vi "Methods to Method Info.vi"(10 "Class":string, 11 "Methods from Node":T2(array[cluster])) -> (2 "Methods for Tree":T1(array[cluster]), 3 "Methods[]":T3(array[cluster]))   [LabVIEW 2023] (continued)
"Class Name (localized)"="VI"}, "Method Info"={"Unique ID string"="42a", "Data name"="Transaction.Fail", "Short name (localized)"="Transaction.Fail", "Long name (localized)"="Transaction:Fail"}, "Method Flags"={"IsDeprecated"=FALSE, "IsPrivate"=FALSE, "IsScripting"=TRUE, "IsNotInRun-Time"=TRUE}, "Divider"=FALSE}, {"Class Info"={"Unique ID string"="2", "Parent ID string"="", "Class Name (unlocalized)"="VI", "Class Name (localized)"="VI"}, "Method Info"={"Unique ID string"="42b", "Data name"="VI Strings.Export Private", "Short name (localized)"="VI Strings.Export Private", "Long name (localized)"="VI Strings:Export Private"}, "Method Flags"={"IsDeprecated"=FALSE, "IsPrivate"=TRUE, "IsScripting"=FALSE, "IsNotInRun-Time"=TRUE}, "Divider"=FALSE}, {"Class Info"={"Unique ID string"="2", "Parent ID string"="", "Class Name (unlocalized)"="VI", "Class Name (localized)"="VI"}, "Method Info"={"Unique ID string"="42c", "Data name"="BD.Get Image Scaled", "Short name (localized)"="BD.Get Image Scaled", "Long name (localized)"="Block Diagram:Get Image Scaled"}, "Method Flags"={"IsDeprecated"=FALSE, "IsPrivate"=FALSE, "IsScripting"=FALSE, "IsNotInRun-Time"=TRUE}, "Divider"=FALSE}, {"Class Info"={"Unique ID string"="2", "Parent ID string"="", "Class Name (unlocalized)"="VI", "Class Name (localized)"="VI"}, "Method Info"={"Unique ID string"="42d", "Data name"="Get Conpane Image", "Short name (localized)"="Get Conpane Image", "Long name (localized)"="Get Conpane Image"}, "Method Flags"={"IsDeprecated"=FALSE, "IsPrivate"=FALSE, "IsScripting"=TRUE, "IsNotInRun-Time"=FALSE}, "Divider"=FALSE}, {"Class Info"={"Unique ID string"="2", "Parent ID string"="", "Class Name (unlocalized)"="VI", "Class Name (localized)"="VI"}, "Method Info"={"Unique ID string"="42e", "Data name"="RP.Lock Control", "Short name (localized)"="RP.Lock Control", "Long name (localized)"="Remote Panel:Lock Control"}, "Method Flags"={"IsDeprecated"=FALSE, "IsPrivate"=FALSE, "IsScripting"=FALSE, "IsNotInRun-Time"=FALSE}, "Divider"=FALSE}, {"Class Info"={"Unique ID string"="2", "Parent ID string"="", "Class Name (unlocalized)"="VI", "Class Name (localized)"="VI"}, "Method Info"={"Unique ID string"="42f", "Data name"="RP.Unlock Control", "Short name (localized)"="RP.Unlock Control", "Long name (localized)"="Remote Panel:Unlock Control"}, "Method Flags"={"IsDeprecated"=FALSE, "IsPrivate"=FALSE, "IsScripting"=FALSE, "IsNotInRun-Time"=FALSE}, "Divider"=FALSE}, {"Class Info"={"Unique ID string"="2", "Parent ID string"="", "Class Name (unlocalized)"="VI", "Class Name (localized)"="VI"}, "Method Info"={"Unique ID string"="430", "Data name"="RP.Client Connections", "Short name (localized)"="RP.Client Connections", "Long name (localized)"="Remote Panel:Client Connections"}, "Method Flags"={"IsDeprecated"=FALSE, "IsPrivate"=FALSE, "IsScripting"=FALSE, "IsNotInRun-Time"=FALSE}, "Divider"=FALSE}, {"Class Info"={"Unique ID string"="2", "Parent ID string"="", "Class Name (unlocalized)"="VI", "Class Name (localized)"="VI"}, "Method Info"={"Unique ID string"="431", "Data name"="RP.Close Connection To Client", "Short name (localized)"="RP.Close Connection To Client", "Long name (localized)"="Remote Panel:Close Connection To Client"}, "Method Flags"={"IsDeprecated"=FALSE, "IsPrivate"=FALSE, "IsScripting"=FALSE, "IsNotInRun-Time"=FALSE}, "Divider"=FALSE}, {"Class Info"={"Unique ID string"="2", "Parent ID string"="", "Class Name (unlocalized)"="VI", "Class Name (localized)"="VI"}, "Method Info"={"Unique ID string"="432", "Data name"="User Edits.Allow", "Short name (localized)"="User Edits.Allow", "Long name (localized)"="User Edits:Allow"}, "Method Flags"={"IsDeprecated"=FALSE, "IsPrivate"=TRUE, "IsScripting"=FALSE, "IsNotInRun-Time"=FALSE}, "Divider"=FALSE}, {"Class Info"={"Unique ID string"="2", "Parent ID string"="", "Class Name (unlocalized)"="VI", "Class Name (localized)"="VI"}, "Method Info"={"Unique ID string"="433", "Data name"="User Edits.Block", "Short name (localized)"="User Edits.Block", "Long name (localized)"="User Edits:Block"}, "Method Flags"={"IsDeprecated"=FALSE, "IsPrivate"=TRUE, "IsScripting"=FALSE, "IsNotInRun-Time"=FALSE}, "Divider"=FALSE}, {"Class Info"={"Unique ID string"="2", "Parent ID string"="", "Class Name (unlocalized)"="VI", "Class Name (localized)"="VI"}, "Method Info"={"Unique ID string"="434", "Data name"="FP.Set Close If Lonely", "Short name (localized)"="FP.Set Close If Lonely", "Long name (localized)"="Front Panel:Set Close If Lonely"}, "Method Flags"={"IsDeprecated"=FALSE, "IsPrivate"=TRUE, "IsScripting"=TRUE, "IsNotInRun-Time"=FALSE}, "Divider"=FALSE}, {"Class Info"={"Unique ID string"="2", "Parent ID string"="", "Class Name (unlocalized)"="VI", "Class Name (localized)"="VI"}, "Method Info"={"Unique ID string"="435", "Data name"="VI Hier.Get User GUID", "Short name (localized)"="VI Hier.Get User GUID", "Long name (localized)"="VI Hierarchy:Get User GUID"}, "Method Flags"={"IsDeprecated"=FALSE, "IsPrivate"=TRUE, "IsScripting"=FALSE, "IsNotInRun-Time"=FALSE}, "Divider"=FALSE}, {"Class Info"={"Unique ID string"="2", "Parent ID string"="", "Class Name (unlocalized)"="VI", "Class Name (localized)"="VI"}, "Method Info"={"Unique ID string"="437", "Data name"="Cause Type Propagation", "Short name (localized)"="Cause Type Propagation", "Long name (localized)"="Cause Type Propagation"}, "Method Flags"={"IsDeprecated"=FALSE, "IsPrivate"=TRUE, "IsScripting"=TRUE, "IsNotInRun-Time"=FALSE}, "Divider"=FALSE}, {"Class Info"={"Unique ID string"="2", "Parent ID string"="", "Class Name (unlocalized)"="VI", "Class Name (localized)"="VI"}, "Method Info"={"Unique ID string"="438", "Data name"="FP.Open", "Short name (localized)"="FP.Open", "Long name (localized)"="Front Panel:Open"}, "Method Flags"={"IsDeprecated"=FALSE, "IsPrivate"=FALSE, "IsScripting"=FALSE, "IsNotInRun-Time"=FALSE}, "Divider"=FALSE}, {"Class Info"={"Unique ID string"="2", "Parent ID string"="", "Class Name (unlocalized)"="VI", "Class Name (localized)"="VI"}, "Method Info"={"Unique ID string"="439", "Data name"="BD.Set Mod", "Short name (localized)"="BD.Set Mod", "Long name (localized)"="Block Diagram:Set Mod"}, "Method Flags"={"IsDeprecated"=FALSE, "IsPrivate"=TRUE, "IsScripting"=FALSE, "IsNotInRun-Time"=TRUE}, "Divider"=FALSE}, {"Class Info"={"Unique ID string"="2", "Parent ID string"="", "Class Name (unlocalized)"="VI", "Class Name (localized)"="VI"}, "Method Info"={"Unique ID string"="43a", "Data name"="FP.Set Mod", "Short name (localized)"="FP.Set Mod", "Long name (localized)"="Front Panel:Set Mod"}, "Method Flags"={"IsDeprecated"=FALSE, "IsPrivate"=TRUE, "IsScripting"=FALSE, "IsNotInRun-Time"=TRUE}, "Divider"=FALSE}, {"Class Info"={"Unique ID string"="2", "Parent ID string"="", "Class Name (unlocalized)"="VI", "Class Name (localized)"="VI"}, "Method Info"={"Unique ID string"="43b", "Data name"="Adapt Nodes Private", "Short name (localized)"="Adapt Nodes Private", "Long name (localized)"="Adapt Nodes Private"}, "Method Flags"={"IsDeprecated"=FALSE, "IsPrivate"=TRUE, "IsScripting"=TRUE, "IsNotInRun-Time"=TRUE}, "Divider"=FALSE}, {"Class Info"={"Unique ID string"="2", "Parent ID string"="", "Class Name (unlocalized)"="VI", "Class Name (localized)"="VI"}, "Method Info"={"Unique ID string"="43c", "Data name"="Adapt Nodes", "Short name (localized)"="Adapt Nodes", "Long name (localized)"="Adapt Nodes"}, "Method Flags"={"IsDeprecated"=FALSE, "IsPrivate"=FALSE, "IsScripting"=TRUE, "IsNotInRun-Time"=TRUE}, "Divider"=FALSE}, {"Class Info"={"Unique ID string"="2", "Parent ID string"="", "Class Name (unlocalized)"="VI", "Class Name (localized)"="VI"}, "Method Info"={"Unique ID string"="43e", "Data name"="Synch In All Contexts", "Short name (localized)"="Synch In All Contexts", "Long name (localized)"="Synchronize In All Contexts"}, "Method Flags"={"IsDeprecated"=FALSE, "IsPrivate"=TRUE, "IsScripting"=FALSE, "IsNotInRun-Time"=FALSE}, "Divider"=FALSE}, {"Class Info"={"Unique ID string"="2", "Parent ID string"="", "Class Name (unlocalized)"="VI", "Class Name (localized)"="VI"}, "Method Info"={"Unique ID string"="43f", "Data name"="Enter Text", "Short name (localized)"="Enter Text", "Long name (localized)"="Enter Text"}, "Method Flags"={"IsDeprecated"=FALSE, "IsPrivate"=TRUE, "IsScripting"=FALSE, "IsNotInRun-Time"=FALSE}, "Divider"=FALSE}, {"Class Info"={"Unique ID string"="2", "Parent ID string"="", "Class Name (unlocalized)"="VI", "Class Name (localized)"="VI"}, "Method Info"={"Unique ID string"="440", "Data name"="Gen C Code Variant", "Short name (localized)"="Gen C Code Variant", "Long name (localized)"="Generate C Code Variant"}, "Method Flags"={"IsDeprecated"=FALSE, "IsPrivate"=TRUE, "IsScripting"=FALSE, "IsNotInRun-Time"=FALSE}, "Divider"=FALSE}, {"Class Info"={"Unique ID string"="2", "Parent ID string"="", "Class Name (unlocalized)"="VI", "Class Name (localized)"="VI"}, "Method Info"={"Unique ID string"="441", "Data name"="FP.Center", "Short name (localized)"="FP.Center", "Long name (localized)"="Front Panel:Center"}, "Method Flags"={"IsDeprecated"=FALSE, "IsPrivate"=FALSE, "IsScripting"=FALSE, "IsNotInRun-Time"=FALSE}, "Divider"=FALSE}, {"Class Info"={"Unique ID string"="2", "Parent ID string"="", "Class Name (unlocalized)"="VI", "Class Name (localized)"="VI"}, "Method Info"={"Unique ID string"="443", "Data name"="Create from Reference", "Short name (localized)"="Create from Reference", "Long name (localized)"="Create from Reference"}, "Method Flags"={"IsDeprecated"=FALSE, "IsPrivate"=FALSE, "IsScripting"=TRUE, "IsNotInRun-Time"=TRUE}, "Divider"=FALSE}, {"Class Info"={"Unique ID string"="2", "Parent ID string"="", "Class Name (unlocalized)"="VI", "Class Name (localized)"="VI"}, "Method Info"={"Unique ID string"="445", "Data name"="FP.Run-Time Pos.Get", "Short name (localized)"="FP.Run-Time Pos.Get", "Long name (localized)"="Front Panel:Run-Time Position:Get Position"}, "Method Flags"={"IsDeprecated"=FALSE, "IsPrivate"=FALSE, "IsScripting"=FALSE, "IsNotInRun-Time"=FALSE}, "Divider"=FALSE}, {"Class Info"={"Unique ID string"="2", "Parent ID string"="", "Class Name (unlocalized)"="VI", "Class Name (localized)"="VI"}, "Method Info"={"Unique ID string"="446", "Data name"="FP.Run-Time Pos.Unchanged", "Short name (localized)"="FP.Run-Time Pos.Unchanged", "Long name (localized)"="Front Panel:Run-Time Position:Unchanged"}, "Method Flags"={"IsDeprecated"=FALSE, "IsPrivate"=FALSE, "IsScripting"=FALSE, "IsNotInRun-Time"=FALSE}, "Divider"=FALSE}, {"Class Info"={"Unique ID string"="2", "Parent ID string"="", "Class Name (unlocalized)"="VI", "Class Name (localized)"="VI"}, "Method Info"={"Unique ID string"="447", "Data name"="FP.Run-Time Position.Centered", "Short name (localized)"="FP.Run-Time Position.Centered", "Long name (localized)"="Front Panel:Run-Time Position:Centered"}, "Method Flags"={"IsDeprecated"=FALSE, "IsPrivate"=FALSE, "IsScripting"=FALSE, "IsNotInRun-Time"=FALSE}, "Divider"=FALSE}, {"Class Info"={"Unique ID string"="2", "Parent ID string"="", "Class Name (unlocalized)"="VI", "Class Name (localized)"="VI"}, "Method Info"={"Unique ID string"="448", "Data name"="FP.Run-Time Position.Maximized", "Short name (localized)"="FP.Run-Time Position.Maximized", "Long name (localized)"="Front Panel:Run-Time Position:Maximized"}, "Method Flags"={"IsDeprecated"=FALSE, "IsPrivate"=FALSE, "IsScripting"=FALSE, "IsNotInRun-Time"=FALSE}, "Divider"=FALSE}, {"Class Info"={"Unique ID string"="2", "Parent ID string"="", "Class Name (unlocalized)"="VI", "Class Name (localized)"="VI"}, "Method Info"={"Unique ID string"="449", "Data name"="FP.Run-Time Position.Minimized", "Short name (localized)"="FP.Run-Time Position.Minimized", "Long name (localized)"="Front Panel:Run-Time Position:Minimized"}, "Method Flags"={"IsDeprecated"=FALSE, "IsPrivate"=FALSE, "IsScripting"=FALSE, "IsNotInRun-Time"=FALSE}, "Divider"=FALSE}, {"Class Info"={"Unique ID string"="2", "Parent ID string"="", "Class Name (unlocalized)"="VI", "Class Name (localized)"="VI"}, "Method Info"={"Unique ID string"="44a", "Data name"="FP.Run-Time Position.Custom", "Short name (localized)"="FP.Run-Time Position.Custom", "Long name (localized)"="Front Panel:Run-Time Position:Custom"}, "Method Flags"={"IsDeprecated"=FALSE, "IsPrivate"=FALSE, "IsScripting"=FALSE, "IsNotInRun-Time"=FALSE}, "Divider"=FALSE}, {"Class Info"={"Unique ID string"="2", "Parent ID string"="", "Class Name (unlocalized)"="VI", "Class Name (localized)"="VI"}, "Method Info"={"Unique ID string"="44b", "Data name"="DisconnectFromLibrary", "Short name (localized)"="DisconnectFromLibrary", "Long name (localized)"="Disconnect From Library"}, "Method Flags"={"IsDeprecated"=FALSE, "IsPrivate"=FALSE, "IsScripting"=FALSE, "IsNotInRun-Time"=TRUE}, "Divider"=FALSE}, {"Class Info"={"Unique ID string"="2", "Parent ID string"="", "Class Name (unlocalized)"="VI", "Class Name (localized)"="VI"}, "Method Info"={"Unique ID string"="44d", "Data name"="Replicate Conpane", "Short name (localized)"="Replicate Conpane", "Long name (localized)"="Replicate Conpane"}, "Method Flags"={"IsDeprecated"=FALSE, "IsPrivate"=FALSE, "IsScripting"=TRUE, "IsNotInRun-Time"=FALSE}, "Divider"=FALSE}, {"Class Info"={"Unique ID string"="2", "Parent ID string"="", "Class Name (unlocalized)"="VI", "Class Name (localized)"="VI"}, "Method Info"={"Unique ID string"="44e", "Data name"="AddASPending", "Short name (localized)"="AddASPending", "Long name (localized)"="Add To AutoSave Pending List"}, "Method Flags"={"IsDeprecated"=FALSE, "IsPrivate"=TRUE, "IsScripting"=FALSE, "IsNotInRun-Time"=TRUE}, "Divider"=FALSE}, {"Class Info"={"Unique ID string"="2", "Parent ID string"="", "Class Name (unlocalized)"="VI", "Class Name (localized)"="VI"}, "Method Info"={"Unique ID string"="44f", "Data name"="RemoveBreakpoints", "Short name (localized)"="RemoveBreakpoints", "Long name (localized)"="Remove Breakpoints"}, "Method Flags"={"IsDeprecated"=FALSE, "IsPrivate"=TRUE, "IsScripting"=TRUE, "IsNotInRun-Time"=FALSE}, "Divider"=FALSE}, {"Class Info"={"Unique ID string"="2", "Parent ID string"="", "Class Name (unlocalized)"="VI", "Class Name (localized)"="VI"}, "Method Info"={"Unique ID string"="451", "Data name"="Save.Instrument(NoSync)", "Short name (localized)"="Save.Instrument(NoSync)", "Long name (localized)"="Save:Instrument (No Sync)"}, "Method Flags"={"IsDeprecated"=FALSE, "IsPrivate"=TRUE, "IsScripting"=FALSE, "IsNotInRun-Time"=TRUE}, "Divider"=FALSE}, {"Class Info"={"Unique ID string"="2", "Parent ID string"="", "Class Name (unlocalized)"="VI", "Class Name (localized)"="VI"}, "Method Info"={"Unique ID string"="452", "Data name"="Get Errors", "Short name (localized)"="Get Errors", "Long name (localized)"="Get Errors"}, "Method Flags"={"IsDeprecated"=FALSE, "IsPrivate"=TRUE, "IsScripting"=TRUE, "IsNotInRun-Time"=FALSE}, "Divider"=FALSE}, {"Class Info"={"Unique ID string"="2", "Parent ID string"="", "Class Name (unlocalized)"="VI", "Class Name (localized)"="VI"}, "Method Info"={"Unique ID string"="453", "Data name"="Tag.Get Tag Names", "Short name (localized)"="Tag.Get Tag Names", "Long name (localized)"="Tag:Get Names"}, "Method Flags"={"IsDeprecated"=FALSE, "IsPrivate"=TRUE, "IsScripting"=FALSE, "IsNotInRun-Time"=FALSE}, "Divider"=FALSE}, {"Class Info"={"Unique ID string"="2", "Parent ID string"="", "Class Name (unlocalized)"="VI", "Class Name (localized)"="VI"}, "Method Info"={"Unique ID string"="454", "Data name"="GiveTemporaryUnsavedName", "Short name (localized)"="GiveTemporaryUnsavedName", "Long name (localized)"="Give Temporary Unsaved Name"}, "Method Flags"={"IsDeprecated"=FALSE, "IsPrivate"=TRUE, "IsScripting"=FALSE, "IsNotInRun-Time"=TRUE}, "Divider"=FALSE}, {"Class Info"={"Unique ID string"="2", "Parent ID string"="", "Class Name (unlocalized)"="VI", "Class Name (localized)"="VI"}, "Method Info"={"Unique ID string"="455", "Data name"="SetOnlineEdit", "Short name (localized)"="SetOnlineEdit", "Long name (localized)"="Set Online Edit"}, "Method Flags"={"IsDeprecated"=FALSE, "IsPrivate"=TRUE, "IsScripting"=FALSE, "IsNotInRun-Time"=FALSE}, "Divider"=FALSE}, {"Class Info"={"Unique ID string"="2", "Parent ID string"="", "Class Name (unlocalized)"="VI", "Class Name (localized)"="VI"}, "Method Info"={"Unique ID string"="457", "Data name"="CtlVIApplyChanges", "Short name (localized)"="CtlVIApplyChanges", "Long name (localized)"="Control VI Apply Changes"}, "Method Flags"={"IsDeprecated"=FALSE, "IsPrivate"=TRUE, "IsScripting"=FALSE, "IsNotInRun-Time"=FALSE}, "Divider"=FALSE}, {"Class Info"={"Unique ID string"="2", "Parent ID string"="", "Class Name (unlocalized)"="VI", "Class Name (localized)"="VI"}, "Method Info"={"Unique ID string"="458", "Data name"="Set Path", "Short name (localized)"="Set Path", "Long name (localized)"="Set Path"}, "Method Flags"={"IsDeprecated"=FALSE, "IsPrivate"=TRUE, "IsScripting"=FALSE, "IsNotInRun-Time"=TRUE}, "Divider"=FALSE}, {"Class Info"={"Unique ID string"="2", "Parent ID string"="", "Class Name (unlocalized)"="VI", "Class Name (localized)"="VI"}, "Method Info"={"Unique ID string"="459", "Data name"="Set Filename", "Short name (localized)"="Set Filename", "Long name (localized)"="Set Filename"}, "Method Flags"={"IsDeprecated"=FALSE, "IsPrivate"=TRUE, "IsScripting"=TRUE, "IsNotInRun-Time"=FALSE}, "Divider"=FALSE}, {"Class Info"={"Unique ID string"="2", "Parent ID string"="", "Class Name (unlocalized)"="VI", "Class Name (localized)"="VI"}, "Method Info"={"Unique ID string"="45a", "Data name"="Save.CopyAsSystem", "Short name (localized)"="Save.CopyAsSystem", "Long name (localized)"="Save:Copy As System"}, "Method Flags"={"IsDeprecated"=FALSE, "IsPrivate"=TRUE, "IsScripting"=TRUE, "IsNotInRun-Time"=FALSE}, "Divider"=FALSE}, {"Class Info"={"Unique ID string"="2", "Parent ID string"="", "Class Name (unlocalized)"="VI", "Class Name (localized)"="VI"}, "Method Info"={"Unique ID string"="45c", "Data name"="Save.Instrument and Callers Debug", "Short name (localized)"="Save.Instrument and Callers Debug", "Long name (localized)"="Save:Instrument and Callers Debug"}, "Method Flags"={"IsDeprecated"=FALSE, "IsPrivate"=TRUE, "IsScripting"=FALSE, "IsNotInRun-Time"=TRUE}, "Divider"=FALSE}, {"Class Info"={"Unique ID string"="2", "Parent ID string"="", "Class Name (unlocalized)"="VI", "Class Name (localized)"="VI"}, "Method Info"={"Unique ID string"="45d", "Data name"="InvokeBuiltinMenuItem (Not Implemented)", "Short name (localized)"="InvokeBuiltinMenuItem (Not Implemented)", "Long name (localized)"="Invoke Built in Menu Item (Not Implemented)"}, "Method Flags"={"IsDeprecated"=FALSE, "IsPrivate"=TRUE, "IsScripting"=FALSE, "IsNotInRun-Time"=FALSE}, "Divider"=FALSE}, {"Class Info"={"Unique ID string"="2", "Parent ID string"="", "Class Name (unlocalized)"="VI", "Class Name (localized)"="VI"}, "Method Info"={"Unique ID string"="45e", "Data name"="BeginScript (Not Implemented)", "Short name (localized)"="BeginScript (Not Implemented)", "Long name (localized)"="Begin Scripting (Not Implemented)"}, "Method Flags"={"IsDeprecated"=FALSE, "IsPrivate"=TRUE, "IsScripting"=TRUE, "IsNotInRun-Time"=FALSE}, "Divider"=FALSE}, {"Class Info"={"Unique ID string"="2", "Parent ID string"="", "Class Name (unlocalized)"="VI", "Class Name (localized)"="VI"}, "Method Info"={"Unique ID string"="45f", "Data name"="EndScript (Not Implemented)", "Short name (localized)"="EndScript (Not Implemented)", "Long name (localized)"="End Scripting (Not Implemented)"}, "Method Flags"={"IsDeprecated"=FALSE, "IsPrivate"=TRUE, "IsScripting"=TRUE, "IsNotInRun-Time"=FALSE}, "Divider"=FALSE}, {"Class Info"={"Unique ID string"="2", "Parent ID string"="", "Class Name (unlocalized)"="VI", "Class Name (localized)"="VI"}, "Method Info"={"Unique ID string"="460", "Data name"="MoveObjects", "Short name (localized)"="MoveObjects", "Long name (localized)"="Move Objects"}, "Method Flags"={"IsDeprecated"=FALSE, "IsPrivate"=FALSE, "IsScripting"=TRUE, "IsNotInRun-Time"=TRUE}, "Divider"=FALSE}, {"Class Info"={"Unique ID string"="2", "Parent ID string"="", "Class Name (unlocalized)"="VI", "Class Name (localized)"="VI"}, "Method Info"={"Unique ID string"="461", "Data name"="GetMenuItemState (Not Implemented)", "Short name (localized)"="GetMenuItemState (Not Implemented)", "Long name (localized)"="Get Menu Item State (Not Implemented)"}, "Method Flags"={"IsDeprecated"=FALSE, "IsPrivate"=TRUE, "IsScripting"=FALSE, "IsNotInRun-Time"=FALSE}, "Divider"=FALSE}, {"Class Info"={"Unique ID string"="2", "Parent ID string"="", "Class Name (unlocalized)"="VI", "Class Name (localized)"="VI"}, "Method Info"={"Unique ID string"="462", "Data name"="SuppressBackup (Not Implemented)", "Short name (localized)"="SuppressBackup (Not Implemented)", "Long name (localized)"="Backup:Suppress (Not Implemented)"}, "Method Flags"={"IsDeprecated"=FALSE, "IsPrivate"=TRUE, "IsScripting"=FALSE, "IsNotInRun-Time"=FALSE}, "Divider"=FALSE}, {"Class Info"={"Unique ID string"="2", "Parent ID string"="", "Class Name (unlocalized)"="VI", "Class Name (localized)"="VI"}, "Method Info"={"Unique ID string"="463", "Data name"="UnsuppressBackup (Not Implemented)", "Short name (localized)"="UnsuppressBackup (Not Implemented)", "Long name (localized)"="Backup:Unsuppress (Not Implemented)"}, "Method Flags"={"IsDeprecated"=FALSE, "IsPrivate"=TRUE, "IsScripting"=FALSE, "IsNotInRun-Time"=FALSE}, "Divider"=FALSE}, {"Class Info"={"Unique ID string"="2", "Parent ID string"="", "Class Name (unlocalized)"="VI", "Class Name (localized)"="VI"}, "Method Info"={"Unique ID string"="464", "Data name"="FindCtrlWithKeyFocus", "Short name (localized)"="FindCtrlWithKeyFocus", "Long name (localized)"="Find Control with Key Focus"}, "Method Flags"={"IsDeprecated"=FALSE, "IsPrivate"=FALSE, "IsScripting"=FALSE, "IsNotInRun-Time"=FALSE}, "Divider"=FALSE}, {"Class Info"={"Unique ID string"="2", "Parent ID string"="", "Class Name (unlocalized)"="VI", "Class Name (localized)"="VI"}, "Method Info"={"Unique ID string"="465", "Data name"="SetVIMod", "Short name (localized)"="SetVIMod", "Long name (localized)"="Set VI Mod"}, "Method Flags"={"IsDeprecated"=FALSE, "IsPrivate"=TRUE, "IsScripting"=FALSE, "IsNotInRun-Time"=TRUE}, "Divider"=FALSE}, {"Class Info"={"Unique ID string"="2", "Parent ID string"="", "Class Name (unlocalized)"="VI", "Class Name (localized)"="VI"}, "Method Info"={"Unique ID string"="466", "Data name"="Compile", "Short name (localized)"="Compile", "Long name (localized)"="Compile:VI"}, "Method Flags"={"IsDeprecated"=FALSE, "IsPrivate"=FALSE, "IsScripting"=TRUE, "IsNotInRun-Time"=FALSE}, "Divider"=FALSE}, {"Class Info"={"Unique ID string"="2", "Parent ID string"="", "Class Name (unlocalized)"="VI", "Class Name (localized)"="VI"}, "Method Info"={"Unique ID string"="467", "Data name"="Run VI And Deploy", "Short name (localized)"="Run VI And Deploy", "Long name (localized)"="Run VI And Deploy"}, "Method Flags"={"IsDeprecated"=FALSE, "IsPrivate"=TRUE, "IsScripting"=FALSE, "IsNotInRun-Time"=FALSE}, "Divider"=FALSE}, {"Class Info"={"Unique ID string"="2", "Parent ID string"="", "Class Name (unlocalized)"="VI", "Class Name (localized)"="VI"}, "Method Info"={"Unique ID string"="468", "Data name"="DeployVI", "Short name (localized)"="DeployVI", "Long name (localized)"="Deploy VI"}, "Method Flags"={"IsDeprecated"=FALSE, "IsPrivate"=TRUE, "IsScripting"=FALSE, "IsNotInRun-Time"=FALSE}, "Divider"=FALSE}, {"Class Info"={"Unique ID string"="2", "Parent ID string"="", "Class Name (unlocalized)"="VI", "Class Name (localized)"="VI"}, "Method Info"={"Unique ID string"="469", "Data name"="LadderVIClearLadderEditor", "Short name (localized)"="LadderVIClearLadderEditor", "Long name (localized)"="LadderVI Clear Ladder Editor"}, "Method Flags"={"IsDeprecated"=FALSE, "IsPrivate"=TRUE, "IsScripting"=FALSE, "IsNotInRun-Time"=FALSE}, "Divider"=FALSE}, {"Class Info"={"Unique ID string"="2", "Parent ID string"="", "Class Name (unlocalized)"="VI", "Class Name (localized)"="VI"}, "Method Info"={"Unique ID string"="46a", "Data name"="Ctrl Val.Get Default", "Short name (localized)"="Ctrl Val.Get Default", "Long name (localized)"="Control Value:Get Default"}, "Method Flags"={"IsDeprecated"=FALSE, "IsPrivate"=TRUE, "IsScripting"=FALSE, "IsNotInRun-Time"=FALSE}, "Divider"=FALSE}, {"Class Info"={"Unique ID string"="2", "Parent ID string"="", "Class Name (unlocalized)"="VI", "Class Name (localized)"="VI"}, "Method Info"={"Unique ID string"="46b", "Data name"="Ctrl Val.Get Array Element Default", "Short name (localized)"="Ctrl Val.Get Array Element Default", "Long name (localized)"="Control Value:Get Array Element Default"}, "Method Flags"={"IsDeprecated"=FALSE, "IsPrivate"=TRUE, "IsScripting"=FALSE, "IsNotInRun-Time"=FALSE}, "Divider"=FALSE}, {"Class Info"={"Unique ID string"="2", "Parent ID string"="", "Class Name (unlocalized)"="VI", "Class Name (localized)"="VI"}, "Method Info"={"Unique ID string"="46c", "Data name"="GetNamedInstanceVI", "Short name (localized)"="GetNamedInstanceVI", "Long name (localized)"="Get Named Instance VI"}, "Method Flags"={"IsDeprecated"=FALSE, "IsPrivate"=TRUE, "IsScripting"=FALSE, "IsNotInRun-Time"=FALSE}, "Divider"=FALSE}, {"Class Info"={"Unique ID string"="2", "Parent ID string"="", "Class Name (unlocalized)"="VI", "Class Name (localized)"="VI"}, "Method Info"={"Unique ID string"="46d", "Data name"="CodeCov.Reset", "Short name (localized)"="CodeCov.Reset", "Long name (localized)"="Code Coverage:Reset"}, "Method Flags"={"IsDeprecated"=FALSE, "IsPrivate"=TRUE, "IsScripting"=FALSE, "IsNotInRun-Time"=TRUE}, "Divider"=FALSE}, {"Class Info"={"Unique ID string"="2", "Parent ID string"="", "Class Name (unlocalized)"="VI", "Class Name (localized)"="VI"}, "Method Info"={"Unique ID string"="46e", "Data name"="CodeCov.Percentage", "Short name (localized)"="CodeCov.Percentage", "Long name (localized)"="Code Coverage:Percentage"}, "Method Flags"={"IsDeprecated"=FALSE, "IsPrivate"=TRUE, "IsScripting"=FALSE, "IsNotInRun-Time"=TRUE}, "Divider"=FALSE}, {"Class Info"={"Unique ID string"="2", "Parent ID string"="", "Class Name (unlocalized)"="VI", "Class Name (localized)"="VI"}, "Method Info"={"Unique ID string"="46f", "Data name"="CodeCov.UnrunDiags", "Short name (localized)"="CodeCov.UnrunDiags", "Long name (localized)"="Code Coverage:Uncovered Diagrams"}, "Method Flags"={"IsDeprecated"=FALSE, "IsPrivate"=TRUE, "IsScripting"=FALSE, "IsNotInRun-Time"=TRUE}, "Divider"=FALSE}, {"Class Info"={"Unique ID string"="2", "Parent ID string"="", "Class Name (unlocalized)"="VI", "Class Name (localized)"="VI"}, "Method Info"={"Unique ID string"="470", "Data name"="Ctrl Val.Get Type", "Short name (localized)"="Ctrl Val.Get Type", "Long name (localized)"="Control Value:Get Type"}, "Method Flags"={"IsDeprecated"=FALSE, "IsPrivate"=TRUE, "IsScripting"=FALSE, "IsNotInRun-Time"=FALSE}, "Divider"=FALSE}, {"Class Info"={"Unique ID string"="2", "Parent ID string"="", "Class Name (unlocalized)"="VI", "Class Name (localized)"="VI"}, "Method Info"={"Unique ID string"="471", "Data name"="SaveAsInteractive", "Short name (localized)"="SaveAsInteractive", "Long name (localized)"="Save:Interactive"}, "Method Flags"={"IsDeprecated"=FALSE, "IsPrivate"=TRUE, "IsScripting"=FALSE, "IsNotInRun-Time"=TRUE}, "Divider"=FALSE}, {"Class Info"={"Unique ID string"="2", "Parent ID string"="", "Class Name (unlocalized)"="VI", "Class Name (localized)"="VI"}, "Method Info"={"Unique ID string"="472", "Data name"="Set Is Instance", "Short name (localized)"="Set Is Instance", "Long name (localized)"="Set Is Instance"}, "Method Flags"={"IsDeprecated"=FALSE, "IsPrivate"=TRUE, "IsScripting"=FALSE, "IsNotInRun-Time"=TRUE}, "Divider"=FALSE}, {"Class Info"={"Unique ID string"="2", "Parent ID string"="", "Class Name (unlocalized)"="VI", "Class Name (localized)"="VI"}, "Method Info"={"Unique ID string"="473", "Data name"="RefreshErrWinEntry", "Short name (localized)"="RefreshErrWinEntry", "Long name (localized)"="Refresh Error Window Entry"}, "Method Flags"={"IsDeprecated"=FALSE, "IsPrivate"=TRUE, "IsScripting"=FALSE, "IsNotInRun-Time"=FALSE}, "Divider"=FALSE}, {"Class Info"={"Unique ID string"="2", "Parent ID string"="", "Class Name (unlocalized)"="VI", "Class Name (localized)"="VI"}, "Method Info"={"Unique ID string"="474", "Data name"="BD.CleanUp", "Short name (localized)"="BD.CleanUp", "Long name (localized)"="Block Diagram:Clean Up"}, "Method Flags"={"IsDeprecated"=FALSE, "IsPrivate"=FALSE, "IsScripting"=FALSE, "IsNotInRun-Time"=FALSE}, "Divider"=FALSE}, {"Class Info"={"Unique ID string"="2", "Parent ID string"="", "Class Name (unlocalized)"="VI", "Class Name (localized)"="VI"}, "Method Info"={"Unique ID string"="477", "Data name"="FP.OpenInNativeWind", "Short name (localized)"="FP.OpenInNativeWind", "Long name (localized)"="Front Panel:Open In Native Window"}, "Method Flags"={"IsDeprecated"=FALSE, "IsPrivate"=TRUE, "IsScripting"=FALSE, "IsNotInRun-Time"=FALSE}, "Divider"=FALSE}, {"Class Info"={"Unique ID string"="2", "Parent ID string"="", "Class Name (unlocalized)"="VI", "Class Name (localized)"="VI"}, "Method Info"={"Unique ID string"="478", "Data name"="BD.OpenInNativeWind", "Short name (localized)"="BD.OpenInNativeWind", "Long name (localized)"="Block Diagram:Open In Native Window"}, "Method Flags"={"IsDeprecated"=FALSE, "IsPrivate"=TRUE, "IsScripting"=FALSE, "IsNotInRun-Time"=FALSE}, "Divider"=FALSE}, {"Class Info"={"Unique ID string"="2", "Parent ID string"="", "Class Name (unlocalized)"="VI", "Class Name (localized)"="VI"}, "Method Info"={"Unique ID string"="479", "Data name"="Detect Parallel Loops", "Short name (localized)"="Detect Parallel Loops", "Long name (localized)"="Detect Parallel Loops"}, "Method Flags"={"IsDeprecated"=FALSE, "IsPrivate"=FALSE, "IsScripting"=FALSE, "IsNotInRun-Time"=TRUE}, "Divider"=FALSE}, {"Class Info"={"Unique ID string"="2", "Parent ID string"="", "Class Name (unlocalized)"="VI", "Class Name (localized)"="VI"}, "Method Info"={"Unique ID string"="47a", "Data name"="Get VI Dependencies", "Short name (localized)"="Get VI Dependencies", "Long name (localized)"="Get VI Dependencies (Names and Paths)"}, "Method Flags"={"IsDeprecated"=FALSE, "IsPrivate"=FALSE, "IsScripting"=FALSE, "IsNotInRun-Time"=FALSE}, "Divider"=FALSE}, {"Class Info"={"Unique ID string"="2", "Parent ID string"="", "Class Name (unlocalized)"="VI", "Class Name (localized)"="VI"}, "Method Info"={"Unique ID string"="47b", "Data name"="StatechartInstantiateVI", "Short name (localized)"="StatechartInstantiateVI", "Long name (localized)"="State Chart Instantiate VI"}, "Method Flags"={"IsDeprecated"=FALSE, "IsPrivate"=TRUE, "IsScripting"=FALSE, "IsNotInRun-Time"=TRUE}, "Divider"=FALSE}, {"Class Info"={"Unique ID string"="2", "Parent ID string"="", "Class Name (unlocalized)"="VI", "Class Name (localized)"="VI"}, "Method Info"={"Unique ID string"="47c", "Data name"="TransferVICleanupProc", "Short name (localized)"="TransferVICleanupProc", "Long name (localized)"="Transfer VI Cleanup Proc"}, "Method Flags"={"IsDeprecated"=FALSE, "IsPrivate"=TRUE, "IsScripting"=FALSE, "IsNotInRun-Time"=FALSE}, "Divider"=FALSE}, {"Class Info"={"Unique ID string"="2", "Parent ID string"="", "Class Name (unlocalized)"="VI", "Class Name (localized)"="VI"}, "Method Info"={"Unique ID string"="47d", "Data name"="Save.VIHierarchyToFolder", "Short name (localized)"="Save.VIHierarchyToFolder", "Long name (localized)"="Save:VI Hierarchy to Folder"}, "Method Flags"={"IsDeprecated"=FALSE, "IsPrivate"=TRUE, "IsScripting"=FALSE, "IsNotInRun-Time"=TRUE}, "Divider"=FALSE}, {"Class Info"={"Unique ID string"="2", "Parent ID string"="", "Class Name (unlocalized)"="VI", "Class Name (localized)"="VI"}, "Method Info"={"Unique ID string"="47e", "Data name"="Get Previous VI", "Short name (localized)"="Get Previous VI", "Long name (localized)"="Library:Get Previous VI from Library"}, "Method Flags"={"IsDeprecated"=FALSE, "IsPrivate"=TRUE, "IsScripting"=FALSE, "IsNotInRun-Time"=FALSE}, "Divider"=FALSE}, {"Class Info"={"Unique ID string"="2", "Parent ID string"="", "Class Name (unlocalized)"="VI", "Class Name (localized)"="VI"}, "Method Info"={"Unique ID string"="47f", "Data name"="Get Next VI", "Short name (localized)"="Get Next VI", "Long name (localized)"="Library:Get Next VI from Library"}, "Method Flags"={"IsDeprecated"=FALSE, "IsPrivate"=TRUE, "IsScripting"=FALSE, "IsNotInRun-Time"=FALSE}, "Divider"=FALSE}, {"Class Info"={"Unique ID string"="2", "Parent ID string"="", "Class Name (unlocalized)"="VI", "Class Name (localized)"="VI"}, "Method Info"={"Unique ID string"="480", "Data name"="PauseVI", "Short name (localized)"="PauseVI", "Long name (localized)"="Pause VI"}, "Method Flags"={"IsDeprecated"=FALSE, "IsPrivate"=FALSE, "IsScripting"=TRUE, "IsNotInRun-Time"=TRUE}, "Divider"=FALSE}, {"Class Info"={"Unique ID string"="2", "Parent ID string"="", "Class Name (unlocalized)"="VI", "Class Name (localized)"="VI"}, "Method Info"={"Unique ID string"="481", "Data name"="Debugging:StepInto", "Short name (localized)"="Debugging:StepInto", "Long name (localized)"="Debugging:Step Into"}, "Method Flags"={"IsDeprecated"=FALSE, "IsPrivate"=FALSE, "IsScripting"=TRUE, "IsNotInRun-Time"=FALSE}, "Divider"=FALSE}, {"Class Info"={"Unique ID string"="2", "Parent ID string"="", "Class Name (unlocalized)"="VI", "Class Name (localized)"="VI"}, "Method Info"={"Unique ID string"="482", "Data name"="Debugging:StepOver", "Short name (localized)"="Debugging:StepOver", "Long name (localized)"="Debugging:Step Over"}, "Method Flags"={"IsDeprecated"=FALSE, "IsPrivate"=FALSE, "IsScripting"=TRUE, "IsNotInRun-Time"=FALSE}, "Divider"=FALSE}, {"Class Info"={"Unique ID string"="2", "Parent ID string"="", "Class Name (unlocalized)"="VI", "Class Name (localized)"="VI"}, "Method Info"={"Unique ID string"="483", "Data name"="Debugging:StepOut", "Short name (localized)"="Debugging:StepOut", "Long name (localized)"="Debugging:Step Out"}, "Method Flags"={"IsDeprecated"=FALSE, "IsPrivate"=FALSE, "IsScripting"=TRUE, "IsNotInRun-Time"=FALSE}, "Divider"=FALSE}, {"Class Info"={"Unique ID string"="2", "Parent ID string"="", "Class Name (unlocalized)"="VI", "Class Name (localized)"="VI"}, "Method Info"={"Unique ID string"="484", "Data name"="Debugging:GetButtonState", "Short name (localized)"="Debugging:GetButtonState", "Long name (localized)"="Debugging:Get Debug Button Display State"}, "Method Flags"={"IsDeprecated"=FALSE, "IsPrivate"=FALSE, "IsScripting"=TRUE, "IsNotInRun-Time"=FALSE}, "Divider"=FALSE}, {"Class Info"={"Unique ID string"="2", "Parent ID string"="", "Class Name (unlocalized)"="VI", "Class Name (localized)"="VI"}, "Method Info"={"Unique ID string"="485", "Data name"="Copy VI Hierarchy FPGA", "Short name (localized)"="Copy VI Hierarchy FPGA", "Long name (localized)"="Copy VI Hierarchy With FPGA Side Effects"}, "Method Flags"={"IsDeprecated"=FALSE, "IsPrivate"=TRUE, "IsScripting"=FALSE, "IsNotInRun-Time"=TRUE}, "Divider"=FALSE}, {"Class Info"={"Unique ID string"="2", "Parent ID string"="", "Class Name (unlocalized)"="VI", "Class Name (localized)"="VI"}, "Method Info"={"Unique ID string"="486", "Data name"="Remove Generics From VI Hierarchy", "Short name (localized)"="Remove Generics From VI Hierarchy", "Long name (localized)"="VI Hierarchy:Remove Generic From VI Hierarchy"}, "Method Flags"={"IsDeprecated"=FALSE, "IsPrivate"=TRUE, "IsScripting"=TRUE, "IsNotInRun-Time"=TRUE}, "Divider"=FALSE}, {"Class Info"={"Unique ID string"="2", "Parent ID string"="", "Class Name (unlocalized)"="VI", "Class Name (localized)"="VI"}, "Method Info"={"Unique ID string"="488", "Data name"="PrepareForCompileAndSave", "Short name (localized)"="PrepareForCompileAndSave", "Long name (localized)"="Save:Prepare For Compile And Save"}, "Method Flags"={"IsDeprecated"=FALSE, "IsPrivate"=TRUE, "IsScripting"=FALSE, "IsNotInRun-Time"=TRUE}, "Divider"=FALSE}, {"Class Info"={"Unique ID string"="2", "Parent ID string"="", "Class Name (unlocalized)"="VI", "Class Name (localized)"="VI"}, "Method Info"={"Unique ID string"="489", "Data name"="Get Undo State", "Short name (localized)"="Get Undo State", "Long name (localized)"="Transaction:Get Undo State"}, "Method Flags"={"IsDeprecated"=FALSE, "IsPrivate"=FALSE, "IsScripting"=TRUE, "IsNotInRun-Time"=FALSE}, "Divider"=FALSE}, {"Class Info"={"Unique ID string"="2", "Parent ID string"="", "Class Name (unlocalized)"="VI", "Class Name (localized)"="VI"}, "Method Info"={"Unique ID string"="490", "Data name"="Get Redo State", "Short name (localized)"="Get Redo State", "Long name (localized)"="Transaction:Get Redo State"}, "Method Flags"={"IsDeprecated"=FALSE, "IsPrivate"=FALSE, "IsScripting"=TRUE, "IsNotInRun-Time"=FALSE}, "Divider"=FALSE}, {"Class Info"={"Unique ID string"="2", "Parent ID string"="", "Class Name (unlocalized)"="VI", "Class Name (localized)"="VI"}, "Method Info"={"Unique ID string"="491", "Data name"="CompileToDFIRXML (Not Implemented)", "Short name (localized)"="CompileToDFIRXML (Not Implemented)", "Long name (localized)"="Compile:Compile To DFIR XML (Not Implemented)"}, "Method Flags"={"IsDeprecated"=FALSE, "IsPrivate"=TRUE, "IsScripting"=FALSE, "IsNotInRun-Time"=FALSE}, "Divider"=FALSE}, {"Class Info"={"Unique ID string"="2", "Parent ID string"="", "Class Name (unlocalized)"="VI", "Class Name (localized)"="VI"}, "Method Info"={"Unique ID string"="492", "Data name"="ResetGencodeProfileResults", "Short name (localized)"="ResetGencodeProfileResults", "Long name (localized)"="Reset Generated Code Profile Results"}, "Method Flags"={"IsDeprecated"=FALSE, "IsPrivate"=TRUE, "IsScripting"=FALSE, "IsNotInRun-Time"=TRUE}, "Divider"=FALSE}, {"Class Info"={"Unique ID string"="2", "Parent ID string"="", "Class Name (unlocalized)"="VI", "Class Name (localized)"="VI"}, "Method Info"={"Unique ID string"="493", "Data name"="CompileToDFIRCPP", "Short name (localized)"="CompileToDFIRCPP", "Long name (localized)"="Compile:Compile To DFIR CPP"}, "Method Flags"={"IsDeprecated"=FALSE, "IsPrivate"=TRUE, "IsScripting"=FALSE, "IsNotInRun-Time"=TRUE}, "Divider"=FALSE}, {"Class Info"={"Unique ID string"="2", "Parent ID string"="", "Class Name (unlocalized)"="VI", "Class Name (localized)"="VI"}, "Method Info"={"Unique ID string"="494", "Data name"="License.Get License Status", "Short name (localized)"="License.Get License Status", "Long name (localized)"="License:Get License Status"}, "Method Flags"={"IsDeprecated"=FALSE, "IsPrivate"=TRUE, "IsScripting"=FALSE, "IsNotInRun-Time"=FALSE}, "Divider"=FALSE}, {"Class Info"={"Unique ID string"="2", "Parent ID string"="", "Class Name (unlocalized)"="VI", "Class Name (localized)"="VI"}, "Method Info"={"Unique ID string"="495", "Data name"="GetCompileMetrics", "Short name (localized)"="GetCompileMetrics", "Long name (localized)"="Get Compile Metrics"}, "Method Flags"={"IsDeprecated"=FALSE, "IsPrivate"=FALSE, "IsScripting"=FALSE, "IsNotInRun-Time"=FALSE}, "Divider"=FALSE}, {"Class Info"={"Unique ID string"="2", "Parent ID string"="", "Class Name (unlocalized)"="VI", "Class Name (localized)"="VI"}, "Method Info"={"Unique ID string"="496", "Data name"="Set Is Instance No Owner Check", "Short name (localized)"="Set Is Instance No Owner Check", "Long name (localized)"="Set Is Instance No Owner Check"}, "Method Flags"={"IsDeprecated"=FALSE, "IsPrivate"=TRUE, "IsScripting"=FALSE, "IsNotInRun-Time"=TRUE}, "Divider"=FALSE}, {"Class Info"={"Unique ID string"="2", "Parent ID string"="", "Class Name (unlocalized)"="VI", "Class Name (localized)"="VI"}, "Method Info"={"Unique ID string"="49b", "Data name"="Get Library Access Scope", "Short name (localized)"="Get Library Access Scope", "Long name (localized)"="Get Library Access Scope"}, "Method Flags"={"IsDeprecated"=FALSE, "IsPrivate"=FALSE, "IsScripting"=TRUE, "IsNotInRun-Time"=TRUE}, "Divider"=FALSE}, {"Class Info"={"Unique ID string"="2", "Parent ID string"="", "Class Name (unlocalized)"="VI", "Class Name (localized)"="VI"}, "Method Info"={"Unique ID string"="49c", "Data name"="HasLibrary?", "Short name (localized)"="HasLibrary?", "Long name (localized)"="Library:Has Library?"}, "Method Flags"={"IsDeprecated"=FALSE, "IsPrivate"=TRUE, "IsScripting"=FALSE, 
